vi "VS-Globals.vi"() -> ()   [LabVIEW 2020]
panel:
  out "Abort?":bool
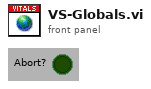
[diagram p1: front panel]
diagram:
